vi "sync_auto_correct.vi"(8 "delay":i32, 9 "threshold":dbl format="%#_13g", 10 "autoVal":cdb[](array[numeric]), 11 "samples":cdb[](array[numeric])) -> (3 "output samples":cdb[](array[numeric]))   [LabVIEW 2014]
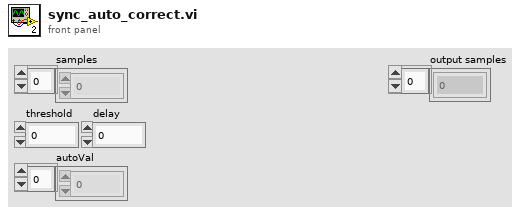
[diagram p1: front panel]
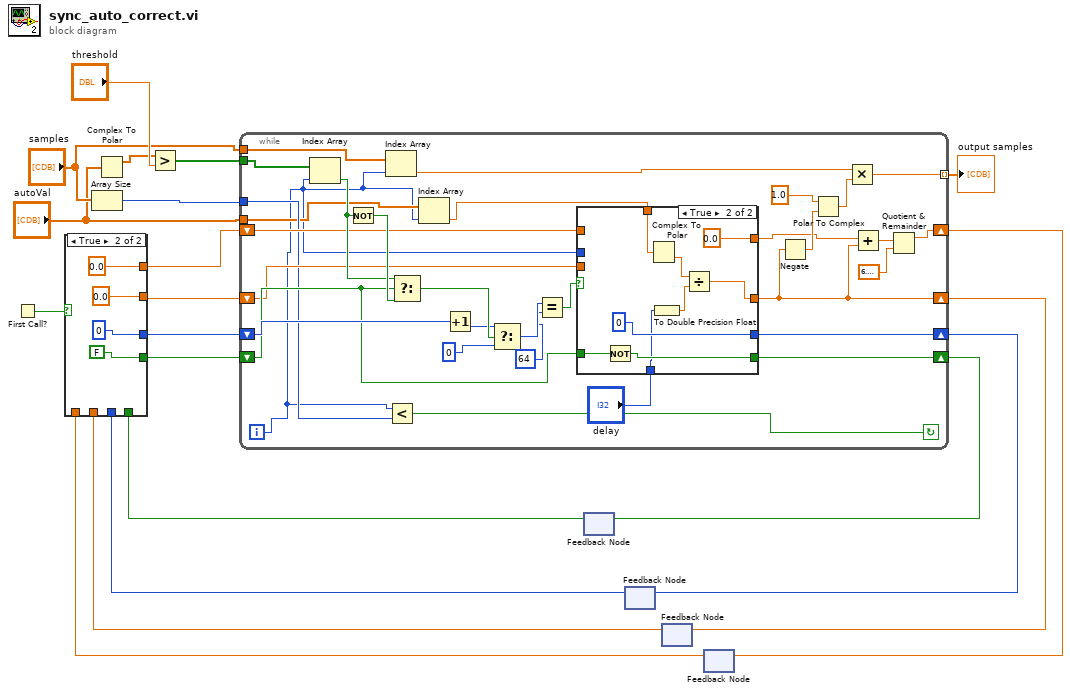
[diagram p0: block diagram]
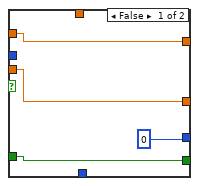
[diagram p3: hidden frame]
diagram:
  n1 = First Call?() -> (First Call?: T/F=w20:bool)
  n2 = Array Size(array="samples") -> (size(s)=w18:i32)
  n3 = Complex To Polar(r * e^(i*theta)="autoVal") -> (r=w13:dbl[])  [unwired: 1 out]
  n4 = Greater?(x=w13, y="threshold") -> (0:w16:bool[])
  n5 = feedback #1() -> (w9:bool)  [unwired: 1 in]
  n6 = feedback #2() -> (w7:i32)  [unwired: 1 in]
  n7 = feedback #3() -> (w5:dbl)  [unwired: 1 in]
  n8 = feedback #4() -> (w3:dbl)  [unwired: 1 in]
  n9 = case shown="True" w20 {
    tunnel: [w22 0.0] -> w19
    tunnel: [w23 0] -> w15
    tunnel: [w24 FALSE] -> w14
    tunnel: [w21 0.0] -> w11
    tunnel: w9 -> [w24 _]
    tunnel: w7 -> [w23 _]
    tunnel: w5 -> [w22 _]
    tunnel: w3 -> [w21 _]
    frame False {
    }
    frame True {
    }
  }
  n10 = while {
    shift-right: [w42] -> w6
    shift-left: w19 -> [w46]
    tunnel: w18 -> [w32]
    tunnel: w16 -> [w59]
    shift-right: [w47] -> w8
    shift-left: w15 -> [w55]
    shift-right: [w48] -> w10
    shift-left: w14 -> [w49]
    tunnel: "samples" -> [w45]
    shift-right: [w35] -> w4
    shift-left: w11 -> [w39]
    tunnel: [w34] -> w12 mode=indexing
    tunnel: "autoVal" -> [w31]
    i -> [w30]
    stop <- w60 continue-if-true
    n11 = Index Array(array=w59, index=w30) -> (element=w57:bool)
    n12 = Not(x=w57) -> (.not. x?=w58:bool)
    n13 = Index Array(array=w45, index=w30) -> (element=w44:cdb)
    n14 = Less?(x=w30, y=w32) -> (x < y?=w60:bool)
    n15 = Select(t=w57, s=w49, f=w58) -> (s? t:f=w56:bool)
    n16 = Index Array(array=w31, index=w30) -> (element=w29:cdb)
    n17 = Increment(x=w55) -> (x+1=w54:i32)
    n18 = Select(t=w54, s=w56, f=0) -> (s? t:f=w52:i32)
    n19 = Equal?(x=w52, y=64) -> (x = y?=w50:bool)
    n20 = case shown="True" w50 {
      tunnel: w49 -> [w64 w73]
      tunnel: [w64 w72] -> w48
      tunnel: [0 0] -> w47
      tunnel: w30 -> [_ _]
      tunnel: "delay" -> [_ w69]
      tunnel: w46 -> [w62 _]
      tunnel: [w62 w66] -> w42
      tunnel: w29 -> [_ w67]
      tunnel: w39 -> [w61 _]
      tunnel: [w61 0.0] -> w38
      frame False {
      }
      frame True {
        n21 = Not(x=w73) -> (.not. x?=w72:bool)
        n22 = Complex To Polar(r * e^(i*theta)=w67) -> (theta=w70:dbl)  [unwired: 1 out]
        n23 = To Double Precision Float(number=w69) -> (double precision float=w68:dbl)
        n24 = Divide(x=w70, y=w68) -> (x/y=w66:dbl)
      }
    }
    n25 = Negate(x=w42) -> (-x=w43:dbl)
    n26 = Polar To Complex(1:w43, 2:1.0) -> (0:w40:cdb)
    n27 = Multiply(x=w44, y=w40) -> (x*y=w34:cdb)
    n28 = Add(x=w38, y=w42) -> (x+y=w37:dbl)
    n29 = Quotient & Remainder(x=w37, y=6.283185307179586) -> (x-y*floor(x/y)=w35:dbl)  [unwired: 1 out]
  }
  "output samples" <- w12
  n30 = feedback-in #1(w10) -> ()
  n31 = feedback-in #2(w8) -> ()
  n32 = feedback-in #3(w6) -> ()
  n33 = feedback-in #4(w4) -> ()
